vi "Load Stim Params.vi"(5 "Stim Parameter Path":path) -> (1 "Right Params":T1, 2 "Left Params":T2)   [LabVIEW 2019]
uses:
  <vilib>/Utility/file.llb/Read Delimited Spreadsheet (I64).vi
panel:
  out "error out":errorcluster
  out "mark after read (chars.)":i32
  out "first row":i64[](array[numeric])
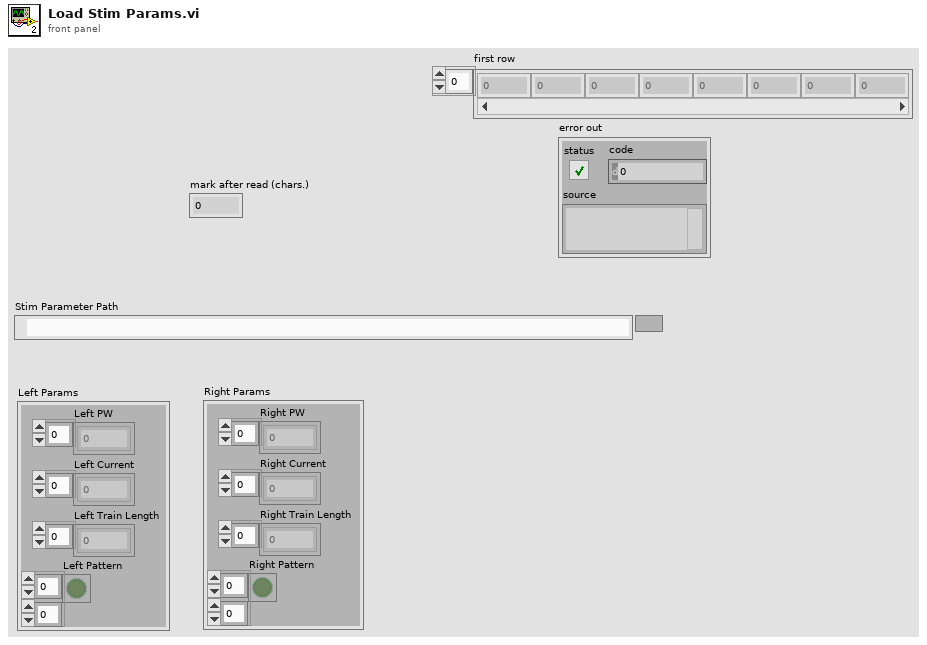
[diagram p1: front panel]
types:
  T1 = cluster{"Right PW":i64[], "Right Current":i64[], "Right Train Length":i64[], "Right Pattern":bool[][]}
  T2 = cluster{"Left PW":i64[], "Left Current":i64[], "Left Train Length":i64[], "Left Pattern":bool[][]}
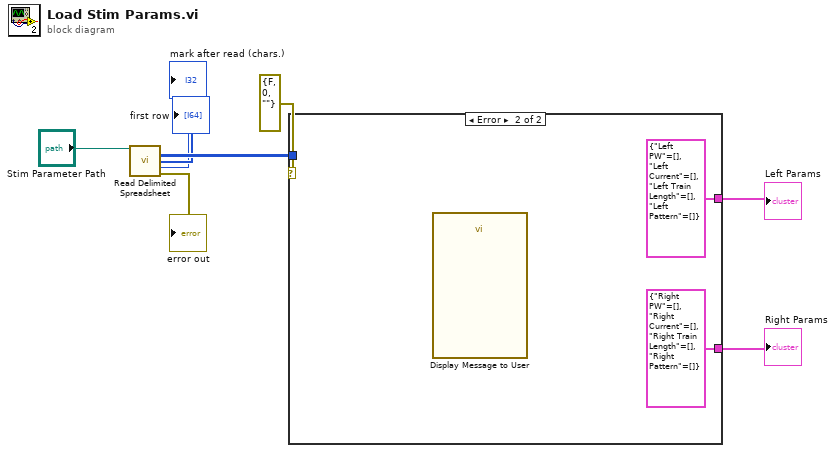
[diagram p0: block diagram]
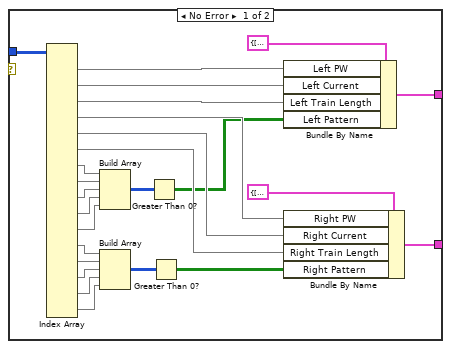
[diagram p2: hidden frame]
diagram:
  n1 = call-poly <vilib>:"Read Delimited Spreadsheet.vi"("file path (dialog if empty)"="Stim Parameter Path") -> ("all rows"=w7:i64[][], "first row"=→"first row":i64[], "mark after read (chars.)"=→"mark after read (chars.)":i32, "error out"=→"error out":errorcluster)  [unwired: 9 in, 2 out]
  n2 = case shown="Error" errorcluster {"status"=FALSE, "code"=0, "source"=""} ("error IO") {
    tunnel: w7 -> [w15 _]
    tunnel: [w14 T2 {"Left PW"=[], "Left Current"=[], "Left Train Length"=[], "Left Pattern"=[]} ("input cluster")] -> w6
    tunnel: [w13 T1 {"Right PW"=[], "Right Current"=[], "Right Train Length"=[], "Right Pattern"=[]} ("input cluster")] -> w5
    frame No Error {
      n3 = Index Array(array=w15) -> (element #1=w28:i64[], element #2=w29:i64[], element #3=w30:i64[], element #4=w31:i64[], element #5=w32:i64[], element #6=w33:i64[], element #7=w27:i64[], element #8=w26:i64[], element #9=w25:i64[], element #10=w24:i64[], element #11=w23:i64[], element #12=w22:i64[], element #13=w21:i64[], element #14=w20:i64[], element #15=w19:i64[], element #16=w18:i64[])  [unwired: 32 in]
      n4 = Build Array(w27, w26, w25, w24, w23) -> (w12:i64[][])
      n5 = Build Array(w22, w21, w20, w19, w18) -> (w10:i64[][])
      n6 = Greater Than 0?(x=w12) -> (x > 0?=w11:bool[][])
      n7 = Greater Than 0?(x=w10) -> (x > 0?=w9:bool[][])
      n8 = Bundle By Name(cluster=T2 {"Left PW"=[], "Left Current"=[], "Left Train Length"=[], "Left Pattern"=[]} ("input cluster"), "Left PW"=w28, "Left Current"=w29, "Left Train Length"=w30, "Left Pattern"=w11) -> (w14:T2)
      n9 = Bundle By Name(cluster=T1 {"Right PW"=[], "Right Current"=[], "Right Train Length"=[], "Right Pattern"=[]} ("input cluster"), "Right PW"=w31, "Right Current"=w32, "Right Train Length"=w33, "Right Pattern"=w9) -> (w13:T1)
    }
    frame Error {
      n10 = call "Display Message to User"() -> ()  [unwired: 10 in, 2 out]
    }
  }
  "Left Params" <- w6
  "Right Params" <- w5
